vi "Kernel.vi"(0 "ref in":refnum<class "G#Template.lvclass">, 1 "object name":string, 2 "option 1":bool, 3 "option 2":bool, 4 "depth":i32, 5 "error in (no error)":errorcluster, 6 "state":T4, 7 "option 3":bool, 8 "attributes in":variant[](array[variant]), 10 "class attributes in":variant[](array[variant])) -> (11 "class attributes out":variant[](array[variant]), 12 "class hierarchy":T1[](array[typedef]), 13 "attributes out":variant[](array[variant]), 14 "ref out":refnum<class "G#Template.lvclass">, 15 "AttributeRefs":u32[](array[numeric]), 16 "static attribute ref":u32, 17 "output 1":bool, 18 "output 2":bool, 19 "error out":errorcluster)   [LabVIEW 2020, in "G#Template.lvclass"]
doc: "Class kernel, creates and destroys the data value references of the class."
uses:
  G#Template.lvclass
  G#Object/utils/G#Object_State.ctl
  C:/ProjectGSharpDevelopment_2020-3/gsharp/VIPM/Files/vi.lib/addons/_AddQ/G#Object/G#Object.lvclass
  G#Object/utils/G#Object_ClassHierarchy.ctl
  protected/ClassAttributes.ctl
  protected/ObjectAttributes.ctl
  ClassAttributesRef.ctl
  ObjectAttributesRef.ctl
  G#Template.lvclass/G#Template.ctl
  G#Object/G#Object.lvclass
panel:
  in  "object attributes type":T2
  in  "class attributes type":T3
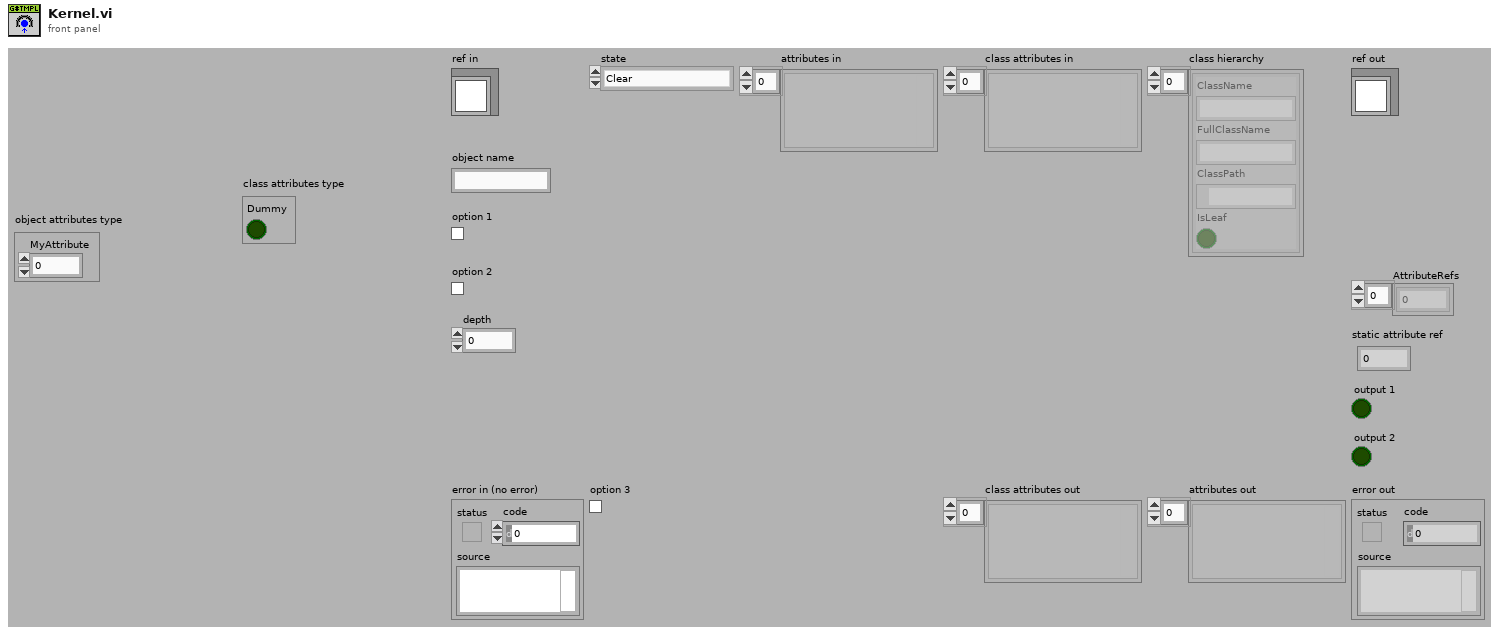
[diagram p1: front panel]
types:
  T1 = typedef "G#Object.lvclass/G#Object_ClassHierarchy.ctl" = cluster{"ClassName":string, "FullClassName":string, "ClassPath":path, "IsLeaf":bool}
  T2 = typedef "G#Template.lvclass/ObjectAttributes.ctl" = cluster{"MyAttribute":dbl}
  T3 = typedef "G#Template.lvclass/ClassAttributes.ctl" = cluster{"Dummy":bool}
  T4 = typedef "G#Object.lvclass/G#Object_State.ctl" = enum16{"Clear", "Create", "Delete", "Get class attributes", "Class hierarchy", "Get attribute value", "Set attribute value"}
  T5 = typedef "G#Template.lvclass/ObjectAttributesRef.ctl" = refnum<data-value>
  T6 = typedef "G#Template.lvclass/ClassAttributesRef.ctl" = refnum<data-value>
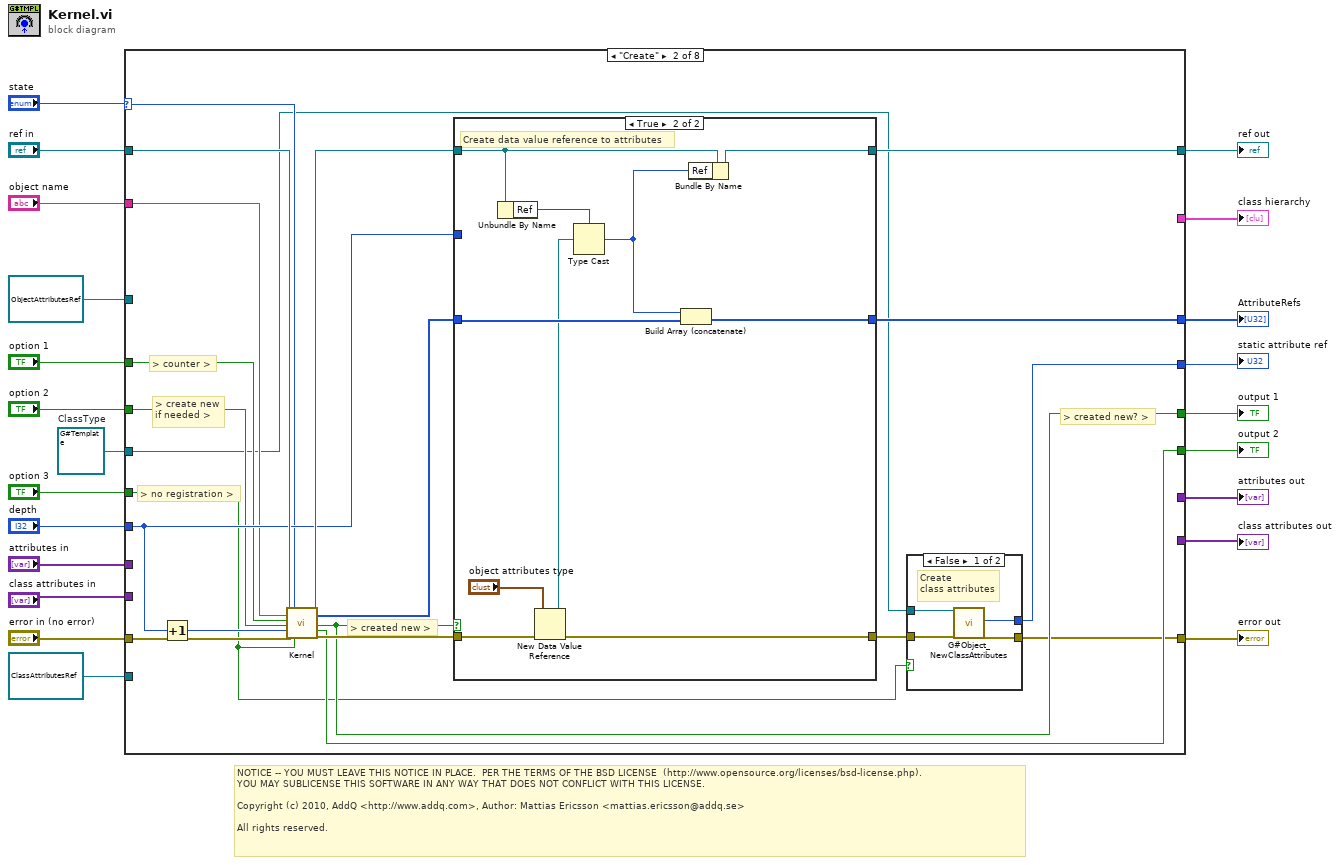
[diagram p0: block diagram]
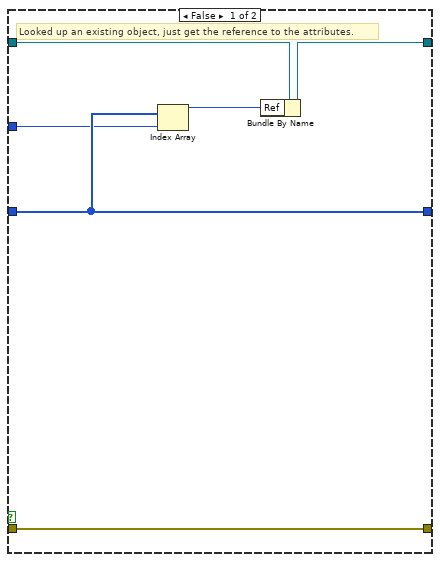
[diagram p4: hidden frame]
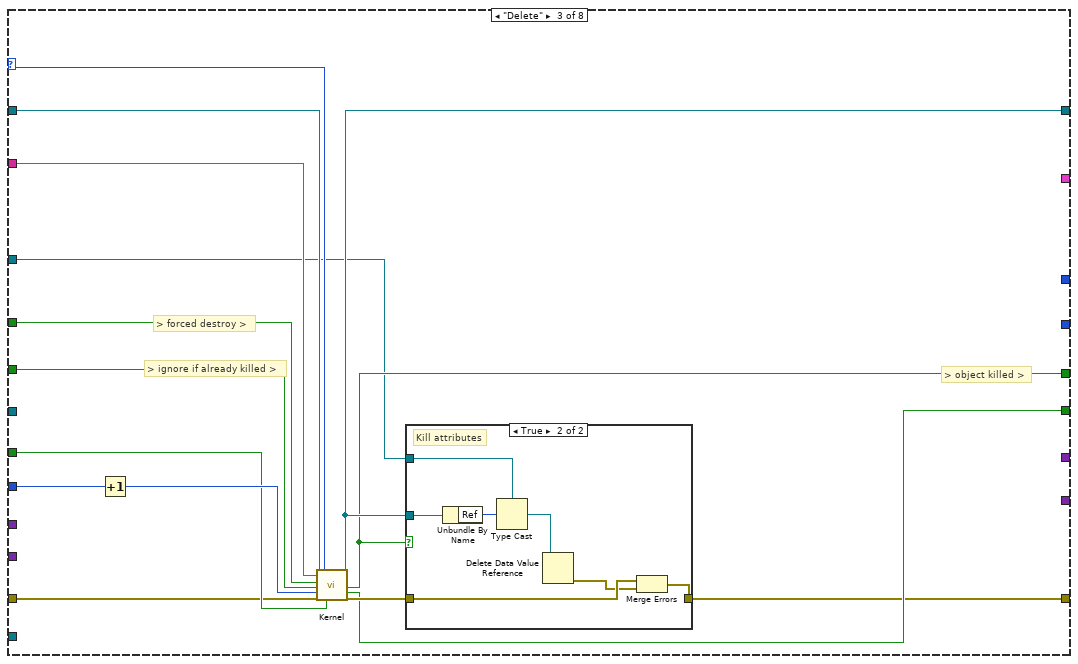
[diagram p5: hidden frame]
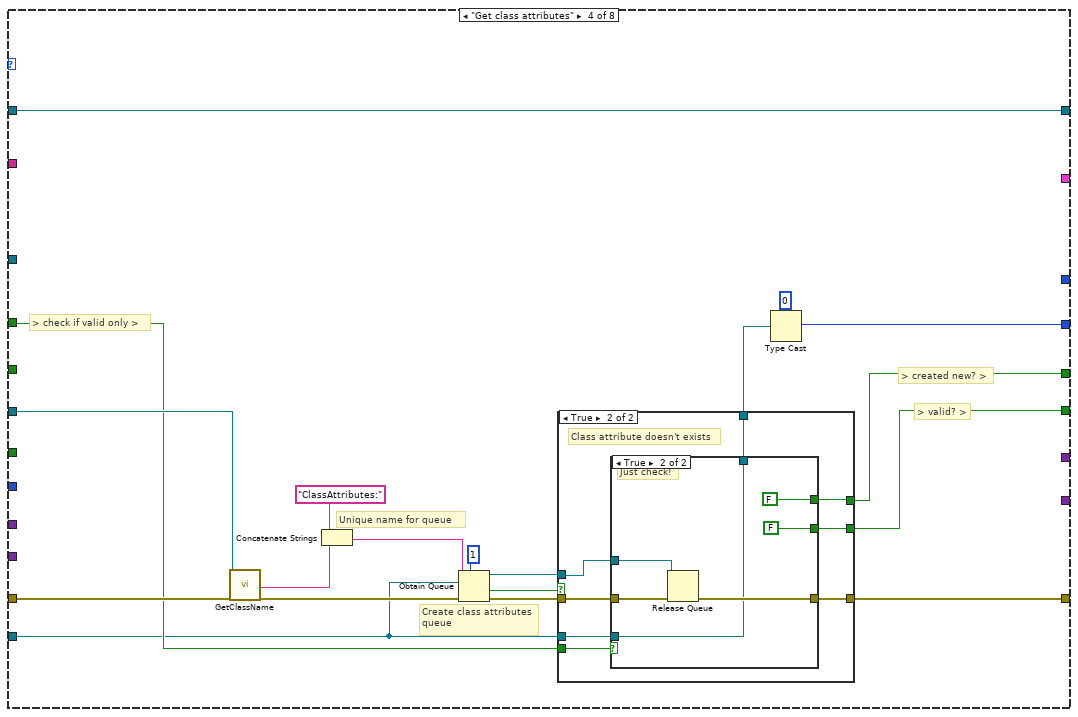
[diagram p7: hidden frame]
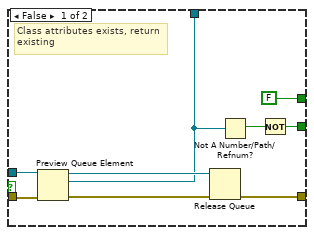
[diagram p8: hidden frame]
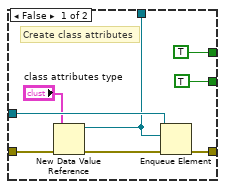
[diagram p9: hidden frame]
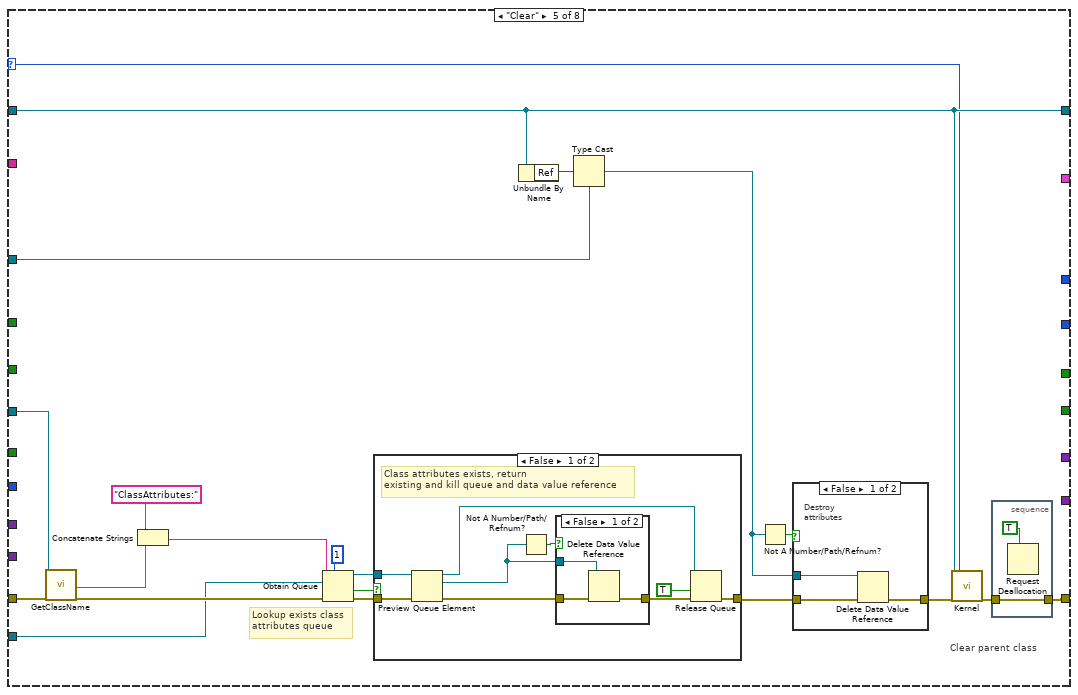
[diagram p10: hidden frame]
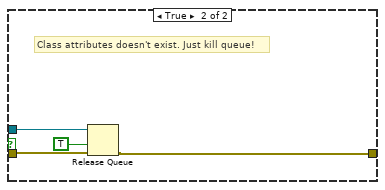
[diagram p13: hidden frame]
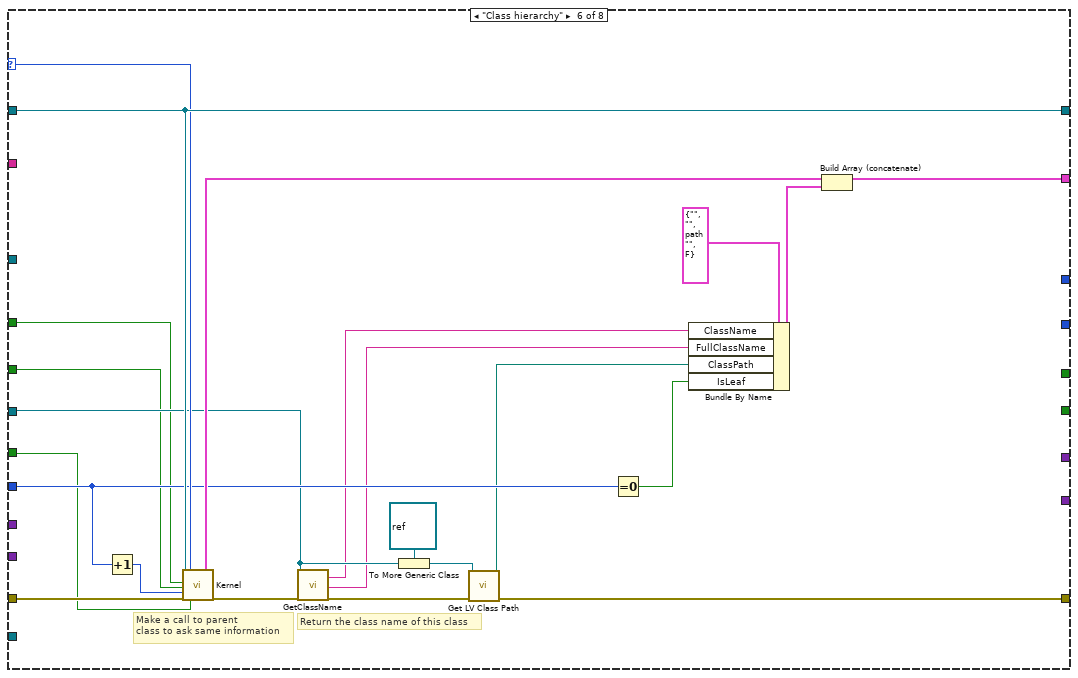
[diagram p14: hidden frame]
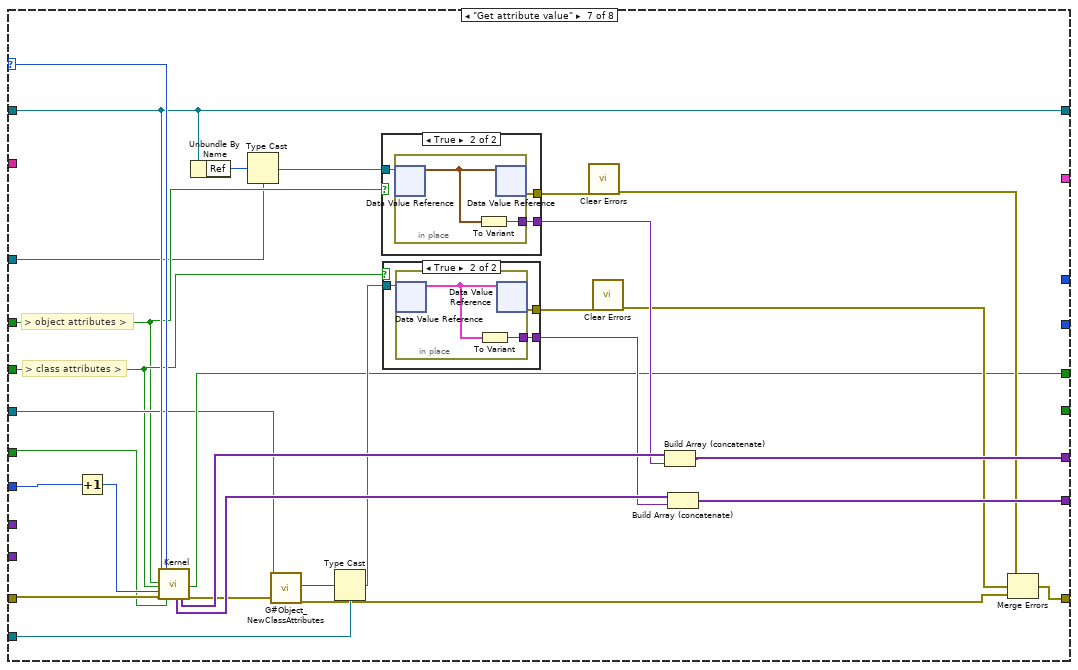
[diagram p15: hidden frame]
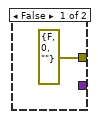
[diagram p16: hidden frame]
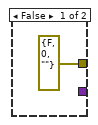
[diagram p17: hidden frame]
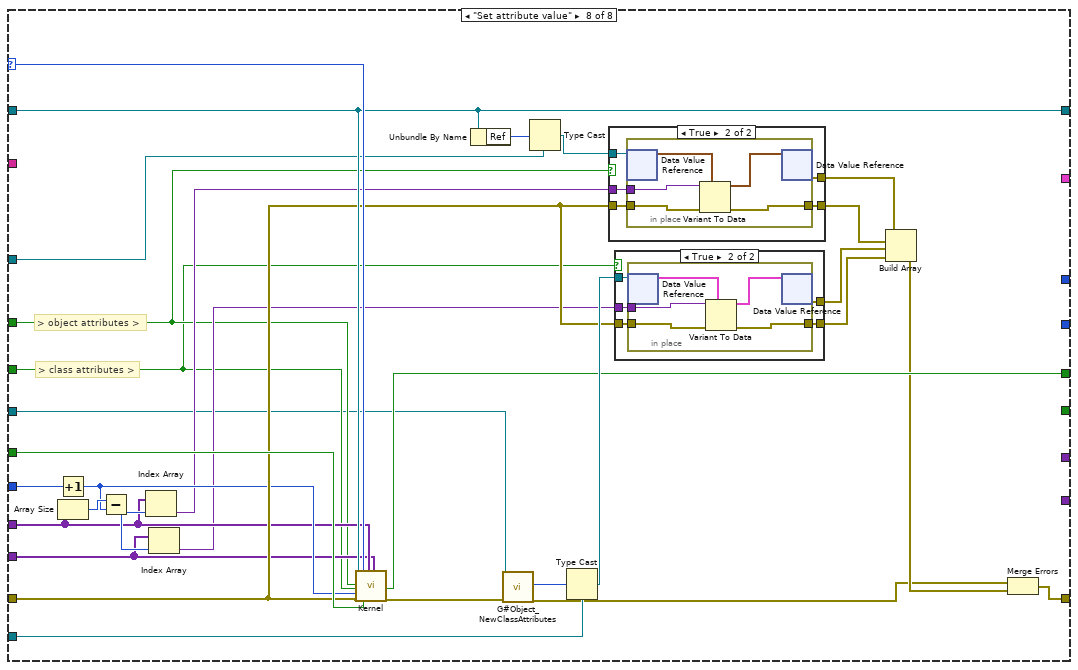
[diagram p18: hidden frame]
diagram:
  w11 = refnum<class "G#Template.lvclass"> refnum  # ClassType
  # "NOTICE -- YOU MUST LEAVE THIS NOTICE IN PLACE.  PER THE TERMS OF THE BSD LICENSE  (http://www.opensource.org/licenses/bsd-license.php).\nYOU MAY SUBLICENSE THIS SOFTWARE IN ANY WAY THAT DOES NOT CONFLICT WITH THIS LICENSE.\n\nCopyright (c) 2010, AddQ <http://www.addq.com>, Author: Mattias Ericsson <mattias.ericsson@addq.se>\n\nAll rights reserved."
  n1 = case shown="\"Create\"" "state" {
    selector: "state" -> [_ w36 w76 _ w146 w202 w233 w275]
    tunnel: "ref in" -> [w24 w41 w73 w107 w147 w203 w227 w274]
    tunnel: [w24 w40 w79 w107 w147 w203 w227 w274] -> w20
    tunnel: "error in (no error)" -> [w23 w39 w68 w106 w159 w188 w232 w268]
    tunnel: [w23 w26 w67 w96 w142 w186 w224 w273] -> w18
    tunnel: "depth" -> [_ w38 w71 _ _ w195 w217 w262]
    tunnel: "object name" -> [_ w37 w69 _ _ _ _ _]
    tunnel: "option 1" -> [_ w35 w77 w92 _ w185 w208 w254]
    tunnel: [_ w34 _ _ _ _ _ _] -> w14
    tunnel: [_ w32 w78 w89 _ _ w214 w269] -> w13
    tunnel: [_ w27 _ w97 _ _ _ _] -> w12
    tunnel: w11 -> [_ w28 _ w94 w150 w191 w211 w251]
    tunnel: T6 refnum ("data value reference") -> [_ _ _ w91 w149 _ w220 w272]
    tunnel: [_ _ _ _ _ w200 _ _] -> w9
    tunnel: [_ _ _ _ _ _ w229 _] -> w8
    tunnel: [_ _ _ _ _ _ w228 _] -> w7
    tunnel: "option 2" -> [_ w31 w75 _ _ w184 w209 w253]
    tunnel: "option 3" -> [_ w25 w70 _ _ w183 w215 w270]
    tunnel: [_ w30 w74 w90 _ _ _ _] -> w4
    tunnel: "attributes in" -> [_ _ _ _ _ _ _ w258]
    tunnel: "class attributes in" -> [_ _ _ _ _ _ _ w255]
    tunnel: T5 refnum ("attributes ref") -> [_ _ w66 _ w140 _ w206 w246]
    frame Default {
    }
    frame "Create" {
      # "> created new >"
      # "> no registration >"
      # "> create new\nif needed >"
      # "> created new? >"
      # "> counter >"
      n2 = Increment(x=w38) -> (x+1=w33:i32)
      n3 = call-parent "Kernel.vi"("reference in"=w41, "object name"=w37, "option 1"=w35, "option 2"=w31, "depth"=w33, "error in (no error)"=w39, "state"=w36, "option 3"=w25) -> ("reference out"=w42:refnum<class "G#Template.lvclass">, "attribute refs"=w43:u32[], "output 1"=w32:bool, "output 2"=w30:bool, "error out"=w44:errorcluster)  [unwired: 3 in, 4 out]
      n4 = case shown="True" w32 {
        tunnel: w44 -> [w55 w65]
        tunnel: [w55 w59] -> w29
        tunnel: w42 -> [w54 w57]
        tunnel: [w53 w60] -> w40
        tunnel: w43 -> [w52 w63]
        tunnel: [w52 w62] -> w34
        tunnel: w38 -> [w51 _]
        frame False {
          # "Looked up an existing object, just get the reference to the attributes."
          n5 = Index Array(array=w52, index=w51) -> (element=w50:u32)
          n6 = Bundle By Name(cluster=w54, "Ref"=w50) -> (w53:refnum<class "G#Template.lvclass">)
        }
        frame True {
          # "Create data value reference to attributes"
          n7 = Unbundle By Name(w57) -> ("Ref"=w56:u32)
          n8 = New Data Value Reference(data value="object attributes type", error in=w65) -> (data value reference=w61:refnum<data-value>, error out=w59:errorcluster)
          n9 = Type Cast(type=w56, x=w61) -> (*(type *) &x=w58:u32)
          n10 = Build Array (concatenate)(w58, w63) -> (w62:u32[])
          n11 = Bundle By Name(cluster=w57, "Ref"=w58) -> (w60:refnum<class "G#Template.lvclass">)
        }
      }
      n12 = case shown="False" w25 {
        tunnel: w29 -> [w48 w49]
        tunnel: w28 -> [w47 _]
        tunnel: [w46 _] -> w27
        tunnel: [w45 w49] -> w26
        frame False {
          # "Create\nclass attributes"
          n13 = call "G#Object_NewClassAttributes.vi"("reference in"=w47, "error in (no error)"=w48) -> ("static attribute ref"=w46:u32, "error out"=w45:errorcluster)  [unwired: 13 in, 3 out]
        }
        frame True {
        }
      }
    }
    frame "Delete" {
      # "> ignore if already killed >"
      # "> object killed >"
      # "> forced destroy >"
      n14 = Increment(x=w71) -> (x+1=w72:i32)
      n15 = call-parent "Kernel.vi"("reference in"=w73, "object name"=w69, "option 1"=w77, "option 2"=w75, "depth"=w72, "error in (no error)"=w68, "state"=w76, "option 3"=w70) -> ("reference out"=w79:refnum<class "G#Template.lvclass">, "output 1"=w78:bool, "output 2"=w74:bool, "error out"=w80:errorcluster)  [unwired: 3 in, 5 out]
      n16 = case shown="True" w78 {
        tunnel: w80 -> [w81 w87]
        tunnel: w79 -> [_ w88]
        tunnel: [w81 w85] -> w67
        tunnel: w66 -> [_ w83]
        frame False {
        }
        frame True {
          # "Kill attributes"
          n17 = Unbundle By Name(w88) -> ("Ref"=w84:u32)
          n18 = Type Cast(type=w83, x=w84) -> (*(type *) &x=w82:T5)
          n19 = Delete Data Value Reference(data value reference=w82) -> (error out=w86:errorcluster)  [unwired: 1 in, 1 out]
          n20 = Merge Errors(w87, w86) -> (w85:errorcluster)
        }
      }
    }
    frame "Get class attributes" {
      # "> valid? >"
      # "> created new? >"
      # "> check if valid only >"
      # "Unique name for queue"
      # "Create class attributes\nqueue"
      n21 = call-dynamic "GetClassName.vi"("reference in"=w94, "error in (no error)"=w106) -> ("full class name"=w95:string, "error out"=w101:errorcluster)  [unwired: 13 in, 3 out]
      n22 = Concatenate Strings("ClassAttributes:" ("string"), w95) -> (w100:string)
      n23 = Obtain Queue(max queue size (-1, unlimited)=1, name (unnamed)=w100, element data type=w91, error in (no error)=w101) -> (queue out=w102:refnum<queue>, created new?=w93:bool, error out=w103:errorcluster)  [unwired: 1 in]
      n24 = case shown="True" w93 {
        tunnel: w103 -> [w116 w124]
        tunnel: w102 -> [w115 w123]
        tunnel: [w114 w121] -> w96
        tunnel: [w110 w122] -> w98
        tunnel: w92 -> [_ w120]
        tunnel: w91 -> [_ w119]
        tunnel: [w109 w118] -> w90
        tunnel: [FALSE w117] -> w89
        frame False {
          # "Class attributes exists, return\nexisting"
          n25 = Preview Queue Element(queue=w115, error in (no error)=w116) -> (queue out=w112:refnum<queue>, element=w110:T6, error out=w113:errorcluster)  [unwired: 1 in, 1 out]
          n26 = Release Queue(queue=w112, error in (no error)=w113) -> (error out=w114:errorcluster)  [unwired: 1 in, 2 out]
          n27 = Not A Number/Path/Refnum?(number/path/refnum=w110) -> (NaN/Path/Refnum?=w108:bool)
          n28 = Not(x=w108) -> (.not. x?=w109:bool)
        }
        frame True {
          # "Class attribute doesn't exists"
          n29 = case shown="True" w120 {
            tunnel: w124 -> [w132 w138]
            tunnel: w123 -> [w130 w137]
            tunnel: [w129 w135] -> w122
            tunnel: [w128 w136] -> w121
            tunnel: w119 -> [_ w135]
            tunnel: [TRUE FALSE] -> w118
            tunnel: [TRUE FALSE] -> w117
            frame False {
              # "Create class attributes"
              n30 = New Data Value Reference(data value="class attributes type", error in=w132) -> (data value reference=w129:refnum<data-value>, error out=w131:errorcluster)
              n31 = Enqueue Element(queue=w130, element=w129, error in (no error)=w131) -> (error out=w128:errorcluster)  [unwired: 1 in, 2 out]
            }
            frame True {
              # "Just check!"
              n32 = Release Queue(queue=w137, error in (no error)=w138) -> (error out=w136:errorcluster)  [unwired: 1 in, 2 out]
            }
          }
        }
      }
      n33 = Type Cast(type=u32 0, x=w98) -> (*(type *) &x=w97:u32)
    }
    frame "Clear" {
      # "Clear parent class"
      # "Lookup exists class\nattributes queue"
      n34 = call-dynamic "GetClassName.vi"("reference in"=w150, "error in (no error)"=w159) -> ("full class name"=w151:string, "error out"=w153:errorcluster)  [unwired: 13 in, 3 out]
      n35 = Concatenate Strings("ClassAttributes:" ("string"), w151) -> (w152:string)
      n36 = Obtain Queue(max queue size (-1, unlimited)=1, name (unnamed)=w152, element data type=w149, error in (no error)=w153) -> (queue out=w154:refnum<queue>, created new?=w155:bool, error out=w156:errorcluster)  [unwired: 1 in]
      n37 = case shown="False" w155 {
        tunnel: w156 -> [w169 w181]
        tunnel: w154 -> [w170 w182]
        tunnel: [w172 w180] -> w145
        frame False {
          # "Class attributes exists, return\nexisting and kill queue and data value reference"
          n38 = Preview Queue Element(queue=w170, error in (no error)=w169) -> (queue out=w167:refnum<queue>, element=w166:T6, error out=w168:errorcluster)  [unwired: 1 in, 1 out]
          n39 = Not A Number/Path/Refnum?(number/path/refnum=w166) -> (NaN/Path/Refnum?=w173:bool)
          n40 = case shown="False" w173 {
            tunnel: w168 -> [w177 w178]
            tunnel: [w176 w178] -> w171
            tunnel: w166 -> [w175 _]
            frame False {
              n41 = Delete Data Value Reference(data value reference=w175, error in=w177) -> (error out=w176:errorcluster)  [unwired: 1 out]
            }
            frame True {
            }
          }
          n42 = Release Queue(queue=w167, force destroy? (F)=TRUE, error in (no error)=w171) -> (error out=w172:errorcluster)  [unwired: 2 out]
        }
        frame True {
          # "Class attributes doesn't exist. Just kill queue!"
          n43 = Release Queue(queue=w182, force destroy? (F)=TRUE, error in (no error)=w181) -> (error out=w180:errorcluster)  [unwired: 2 out]
        }
      }
      n44 = Unbundle By Name(w147) -> ("Ref"=w141:u32)
      n45 = Type Cast(type=w140, x=w141) -> (*(type *) &x=w139:T5)
      n46 = Not A Number/Path/Refnum?(number/path/refnum=w139) -> (NaN/Path/Refnum?=w148:bool)
      n47 = case shown="False" w148 {
        tunnel: w139 -> [w162 _]
        tunnel: w145 -> [w164 w165]
        tunnel: [w163 w165] -> w144
        frame False {
          # "Destroy\nattributes"
          n48 = Delete Data Value Reference(data value reference=w162, error in=w164) -> (error out=w163:errorcluster)  [unwired: 1 out]
        }
        frame True {
        }
      }
      n49 = call-parent "Kernel.vi"("reference in"=w147, "error in (no error)"=w144, "state"=w146) -> ("error out"=w143:errorcluster)  [unwired: 8 in, 8 out]
      n50 = stacked-sequence {
        tunnel: w143 -> [w160]
        tunnel: [w160] -> w142
        frame #0 {
          n51 = Request Deallocation(TRUE ("flag")) -> ()
        }
      }
    }
    frame "Class hierarchy" {
      # "Make a call to parent\nclass to ask same information"
      # "Return the class name of this class"
      n52 = Increment(x=w195) -> (x+1=w196:i32)
      n53 = call-parent "Kernel.vi"("reference in"=w203, "option 1"=w185, "option 2"=w184, "depth"=w196, "error in (no error)"=w188, "state"=w202, "option 3"=w183) -> ("class hierarchy"=w201:T1[], "error out"=w187:errorcluster)  [unwired: 4 in, 7 out]
      n54 = call-dynamic "GetClassName.vi"("reference in"=w191, "error in (no error)"=w187) -> ("class name"=w189:string, "full class name"=w190:string, "error out"=w192:errorcluster)  [unwired: 13 in, 2 out]
      n55 = To More Generic Class(target class=refnum<class> refnum ("object"), reference=w191) -> (generic class reference=w197:refnum<class>)
      n56 = call <vilib>:"Get LV Class Path.vi"("error in (no error)"=w192, "object"=w197) -> ("error out"=w186:errorcluster, "class path"=w193:path)  [unwired: 8 in]
      n57 = Equal To 0?(x=w195) -> (x = 0?=w194:bool)
      n58 = Bundle By Name(cluster=T1 {"ClassName"="", "FullClassName"="", "ClassPath"=path "", "IsLeaf"=FALSE} ("ClassHierarchy"), "ClassName"=w189, "FullClassName"=w190, "ClassPath"=w193, "IsLeaf"=w194) -> (w198:T1)
      n59 = Build Array (concatenate)(w201, w198) -> (w200:T1[])
    }
    frame "Get attribute value" {
      # "> class attributes >"
      # "> object attributes >"
      n60 = Increment(x=w217) -> (x+1=w216:i32)
      n61 = call-parent "Kernel.vi"("reference in"=w227, "option 1"=w208, "option 2"=w209, "depth"=w216, "error in (no error)"=w232, "state"=w233, "option 3"=w215) -> ("class attributes out"=w230:variant[], "attributes out"=w231:variant[], "output 1"=w214:bool, "error out"=w213:errorcluster)  [unwired: 4 in, 5 out]
      n62 = Unbundle By Name(w227) -> ("Ref"=w207:u32)
      n63 = Type Cast(type=w206, x=w207) -> (*(type *) &x=w205:T5)
      n64 = call "G#Object_NewClassAttributes.vi"("reference in"=w211, "error in (no error)"=w213) -> ("static attribute ref"=w210:u32, "error out"=w212:errorcluster)  [unwired: 13 in, 3 out]
      n65 = Type Cast(type=w220, x=w210) -> (*(type *) &x=w219:T6)
      n66 = case shown="True" w208 {
        tunnel: w205 -> [_ w243]
        tunnel: [_ w242] -> w226
        tunnel: [errorcluster {"status"=FALSE, "code"=0, "source"=""} ("error IO") w241] -> w225
        frame False {
        }
        frame True {
          n67 = in-place {
            in-place-border: [w245] -> w242
            n68 = in-place-dvr #1(w243) -> (w244:T2)  [unwired: 1 out]
            n69 = To Variant(anything=w244) -> (Variant=w245:variant)
            n70 = in-place-dvr #1(w244) -> (w241:errorcluster)  [unwired: 1 out]
          }
        }
      }
      n71 = case shown="True" w209 {
        tunnel: [errorcluster {"status"=FALSE, "code"=0, "source"=""} ("error IO") w237] -> w222
        tunnel: w219 -> [_ w236]
        tunnel: [_ w235] -> w218
        frame False {
        }
        frame True {
          n72 = in-place {
            in-place-border: [w239] -> w235
            n73 = in-place-dvr #2(w236) -> (w238:T3)  [unwired: 1 out]
            n74 = To Variant(anything=w238) -> (Variant=w239:variant)
            n75 = in-place-dvr #2(w238) -> (w237:errorcluster)  [unwired: 1 out]
          }
        }
      }
      n76 = call <vilib>:"Clear Errors.vi"("error in (no error)"=w225) -> ("error out"=w223:errorcluster)  [unwired: 5 in, 1 out]
      n77 = call <vilib>:"Clear Errors.vi"("error in (no error)"=w222) -> ("error out"=w221:errorcluster)  [unwired: 5 in, 1 out]
      n78 = Build Array (concatenate)(w231, w226) -> (w229:variant[])
      n79 = Build Array (concatenate)(w230, w218) -> (w228:variant[])
      n80 = Merge Errors(w223, w221, w212) -> (w224:errorcluster)
    }
    frame "Set attribute value" {
      # "> class attributes >"
      # "> object attributes >"
      n81 = Increment(x=w262) -> (x+1=w260:i32)
      n82 = Array Size(array=w258) -> (size(s)=w261:i32)
      n83 = Subtract(x=w261, y=w260) -> (x-y=w259:i32)
      n84 = Index Array(array=w258, index=w259) -> (element=w257:variant)
      n85 = Index Array(array=w255, index=w259) -> (element=w256:variant)
      n86 = call-parent "Kernel.vi"("reference in"=w274, "option 1"=w254, "option 2"=w253, "depth"=w260, "error in (no error)"=w268, "state"=w275, "option 3"=w270, "attributes in"=w258, "class attributes in"=w255) -> ("output 1"=w269:bool, "error out"=w252:errorcluster)  [unwired: 2 in, 7 out]
      n87 = Unbundle By Name(w274) -> ("Ref"=w248:u32)
      n88 = call "G#Object_NewClassAttributes.vi"("reference in"=w251, "error in (no error)"=w252) -> ("static attribute ref"=w250:u32, "error out"=w249:errorcluster)  [unwired: 13 in, 3 out]
      n89 = Type Cast(type=w246, x=w248) -> (*(type *) &x=w247:T5)
      n90 = Type Cast(type=w272, x=w250) -> (*(type *) &x=w271:T6)
      n91 = case shown="True" w254 {
        tunnel: w247 -> [_ w281]
        tunnel: w268 -> [w276 w280]
        tunnel: [w276 w279] -> w267
        tunnel: [w276 w278] -> w266
        tunnel: w257 -> [_ w277]
        frame False {
        }
        frame True {
          n92 = in-place {
            in-place-border: w280 -> [w284]
            in-place-border: [w283] -> w278
            in-place-border: w277 -> [w282]
            n93 = in-place-dvr #3(w281) -> (w286:T2)  [unwired: 1 out]
            n94 = Variant To Data(error in=w284, type=w286, Variant=w282) -> (data=w285:T2, error out=w283:errorcluster)
            n95 = in-place-dvr #3(w285) -> (w279:errorcluster)  [unwired: 1 out]
          }
        }
      }
      n96 = case shown="True" w253 {
        tunnel: w271 -> [_ w292]
        tunnel: w268 -> [w287 w291]
        tunnel: [w287 w290] -> w265
        tunnel: [w287 w289] -> w264
        tunnel: w256 -> [_ w288]
        frame False {
        }
        frame True {
          n97 = in-place {
            in-place-border: w291 -> [w295]
            in-place-border: [w294] -> w289
            in-place-border: w288 -> [w293]
            n98 = in-place-dvr #4(w292) -> (w297:T3)  [unwired: 1 out]
            n99 = Variant To Data(error in=w295, type=w297, Variant=w293) -> (data=w296:T3, error out=w294:errorcluster)
            n100 = in-place-dvr #4(w296) -> (w290:errorcluster)  [unwired: 1 out]
          }
        }
      }
      n101 = Build Array(w267, w266, w265, w264) -> (w263:errorcluster[])
      n102 = Merge Errors(w249, w263) -> (w273:errorcluster)
    }
  }
  "error out" <- w18
  "ref out" <- w20
  "AttributeRefs" <- w14
  "static attribute ref" <- w12
  "output 1" <- w13
  "output 2" <- w4
  "class hierarchy" <- w9
  "attributes out" <- w8
  "class attributes out" <- w7
